vi "Assign Group Transforms.vi"(8 "error in (no error)":errorcluster, 9 "transform in":string, 10 "position":i32, 11 "ParseSVG in":refnum<class "ParseSVG.lvclass">) -> (0 "error out":errorcluster, 1 "transform out":string, 3 "ParseSVG out":refnum<class "ParseSVG.lvclass">)   [LabVIEW 2019, in "ParseSVG.lvclass"]
uses:
  ParseSVG.lvclass
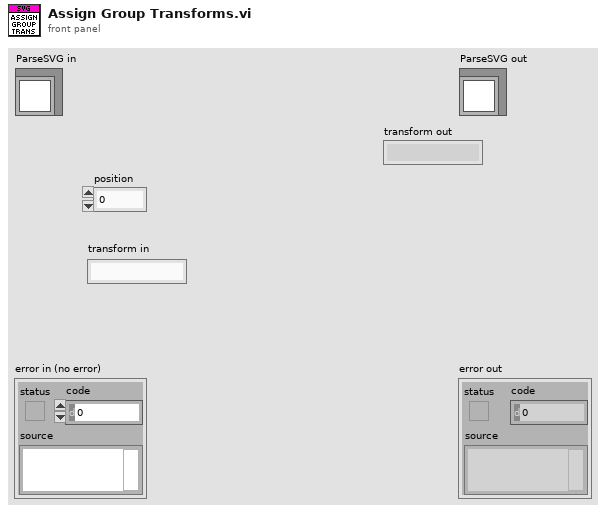
[diagram p1: front panel]
types:
  T1 = cluster{"Start":i32, "id":string, "transforms":string, "End":i32}[]
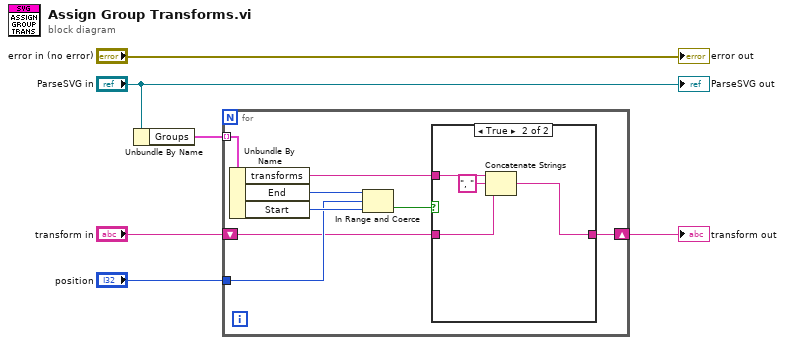
[diagram p0: block diagram]
diagram:
  n1 = Unbundle By Name("ParseSVG in") -> ("Groups"=w4:T1)
  n2 = for {
    tunnel: w4 -> [w14] mode=indexing
    tunnel: "position" -> [w11]
    shift-right: [w7] -> w1
    shift-left: "transform in" -> [w8]
    n3 = Unbundle By Name(w14) -> ("transforms"=w9:string, "End"=w12:i32, "Start"=w13:i32)
    n4 = In Range and Coerce(upper limit=w12, x=w11, lower limit=w13) -> (In Range?=w10:bool)  [unwired: 1 out]
    n5 = case shown="True" w10 {
      tunnel: w9 -> [_ w19]
      tunnel: w8 -> [w15 w16]
      tunnel: [w15 w17] -> w7
      frame False {
      }
      frame True {
        n6 = Concatenate Strings(w19, ", " ("string"), w16) -> (w17:string)
      }
    }
  }
  "transform out" <- w1
  "error out" <- "error in (no error)"
  "ParseSVG out" <- "ParseSVG in"
